vi "Cutting Status.vi"() -> ()   [LabVIEW 2021]
uses:
  Controls/Cutting v0.1.ctl
panel:
  out "Cutting Status":T1
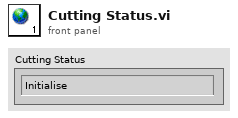
[diagram p1: front panel]
types:
  T1 = typedef "Cutting v0.1.ctl" = enum16{"Initialise", "Clamp Fwd", "Clamp Delay", "Station Fwd", "Station Fwd Delay", "CYL Fwd", "Cut Delay", "CYL Rear", "Wait for Delay", "Station & Clamp Rear", "Done", "Error"}
diagram:
